vi "Main.vi"() -> ()   [LabVIEW 2013]
uses:
  Application Data.ctl
  State.ctl
panel:
  in  "Tahmin":i16
  in  "Tahmin Sayisi":u8=10 min=1
  in  "Tahmin Seç":bool
  out "Mesaj":string
  out "Bitti":bool
  out "Kalan":i16
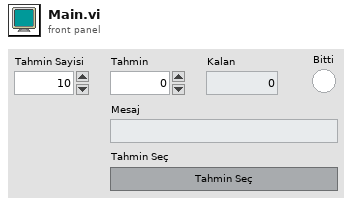
[diagram p1: front panel]
types:
  T1 = typedef "State.ctl" = enum16{"Initialise", "Make Guess", "Wait for event", "Sucess", "Fail", "End"}
  T2 = typedef "Application Data.ctl" = cluster{"Guesses Remaining":u8, "Guess":i16, "Message":string, "Correct":bool}
  T3 = enum8{"Enabled", "Disabled", "Disabled and Grayed Out"}
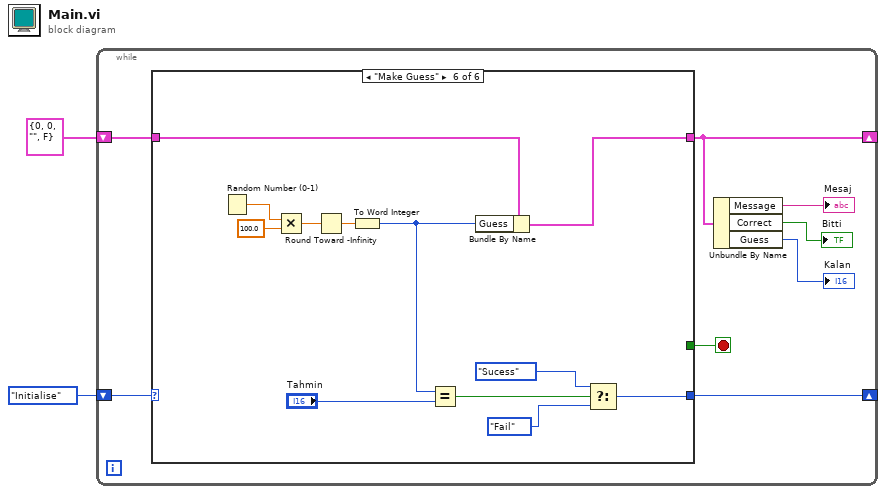
[diagram p0: block diagram]
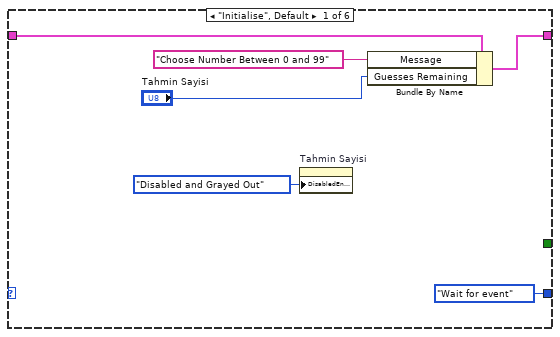
[diagram p2: hidden frame]
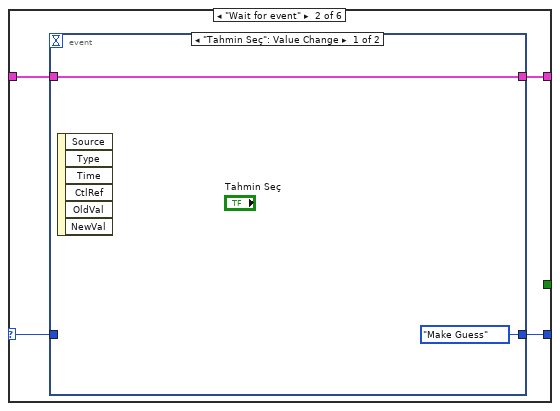
[diagram p3: hidden frame]
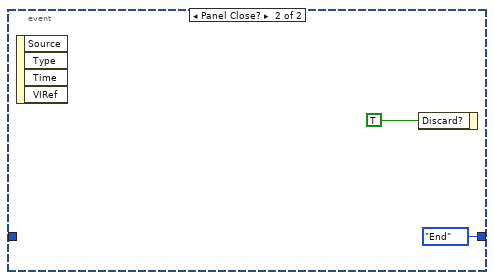
[diagram p4: hidden frame]
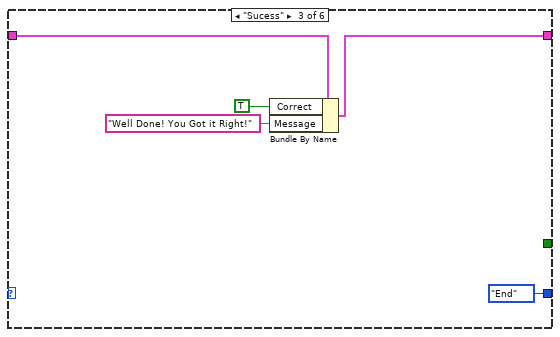
[diagram p5: hidden frame]
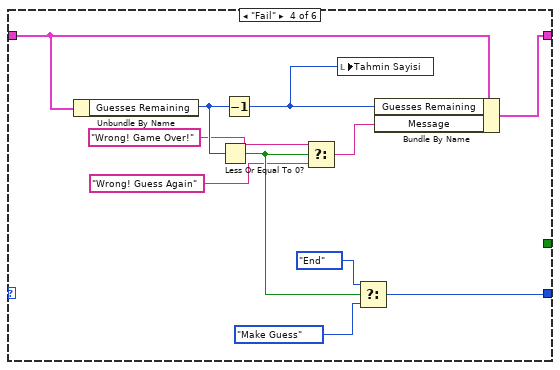
[diagram p6: hidden frame]
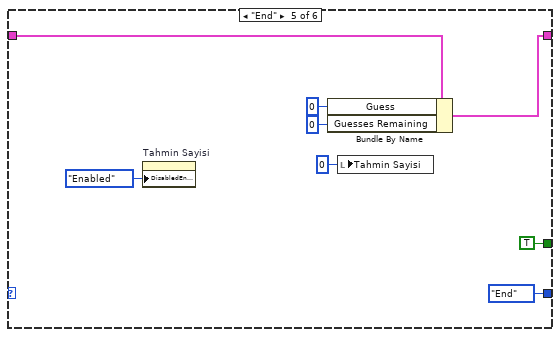
[diagram p7: hidden frame]
diagram:
  n1 = while {
    shift-right: [w9] -> _
    shift-left: T2 {"Guesses Remaining"=0, "Guess"=0, "Message"="", "Correct"=FALSE} ("Application Data") -> [w10]
    shift-right: [w7] -> _
    shift-left: State."Initialise" ("State") -> [w6]
    stop <- w5 stop-if-true
    n2 = case shown="\"Make Guess\"" w6 {
      selector: w6 -> [_ w17 _ _ _ _]
      tunnel: w10 -> [w16 w20 w29 w40 w45 w56]
      tunnel: [w15 w19 w28 w39 w44 w55] -> w9
      tunnel: [State."Wait for event" ("State") w18 State."End" ("State") w37 State."End" ("State") w49] -> w7
      tunnel: [_ _ _ _ TRUE _] -> w5
      frame "Initialise", Default {
        n3 = property on="Tahmin Sayisi" class="DigNum (strict)"("DisabledEnum"=T3."Disabled and Grayed Out" ("Disabled")) -> ()  [unwired: 2 in, 2 out]
        n4 = Bundle By Name(cluster=w16, "Message"="Choose Number Between 0 and 99", "Guesses Remaining"="Tahmin Sayisi") -> (w15:T2)
      }
      frame "Wait for event" {
        n5 = event shown="[0] \"Tahmin Seç\": Value Change" {
          selector: _ -> [_ _]
          dyn-events: _ -> [_ _]
          timeout: _ -> [_ _]
          tunnel: w20 -> [w22 _]
          tunnel: [w22 _] -> w19
          tunnel: [State."Make Guess" ("State") State."End" ("State")] -> w18
          tunnel: w17 -> [_ _]
          event "Tahmin Seç": Value Change {
            n6 = event-data() -> ()  [unwired: 1 in, 6 out]
          }
          event Panel Close? {
            n7 = event-data() -> ()  [unwired: 1 in, 4 out]
            n8 = event-data("Discard?"=TRUE) -> ()  [unwired: 1 in, 1 out]
          }
        }
      }
      frame "Sucess" {
        n9 = Bundle By Name(cluster=w29, "Correct"=TRUE, "Message"="Well Done! You Got it Right!") -> (w28:T2)
      }
      frame "Fail" {
        n10 = Unbundle By Name(w40) -> ("Guesses Remaining"=w38:u8)
        n11 = Less Or Equal To 0?(x=w38) -> (x <= 0?=w34:bool)
        n12 = Decrement(x=w38) -> (x-1=w30:u8)
        n13 = Select(t="Wrong! Game Over!", s=w34, f="Wrong! Guess Again") -> (s? t:f=w31:string)
        n14 = local write "Tahmin Sayisi"(w30) -> ()
        n15 = Select(t=State."End" ("State"), s=w34, f=State."Make Guess" ("State")) -> (s? t:f=w37:T1)
        n16 = Bundle By Name(cluster=w40, "Guesses Remaining"=w30, "Message"=w31) -> (w39:T2)
      }
      frame "End" {
        n17 = property on="Tahmin Sayisi" class="DigNum (strict)"("DisabledEnum"=T3."Enabled" ("Disabled")) -> ()  [unwired: 2 in, 2 out]
        n18 = Bundle By Name(cluster=w45, "Guess"=i16 0, "Guesses Remaining"=u8 0) -> (w44:T2)
        n19 = local write "Tahmin Sayisi"(u8 0 ("Tahmin Sayisi")) -> ()
      }
      frame "Make Guess" {
        n20 = Random Number (0-1)() -> (number: 0 to 1=w59:dbl)
        n21 = Multiply(x=w59, y=100.0) -> (x*y=w60:dbl)
        n22 = Round Toward -Infinity(1:w60) -> (0:w58:dbl)
        n23 = To Word Integer(number=w58) -> (16bit integer=w50:i16)
        n24 = Equal?(x=w50, y="Tahmin") -> (x = y?=w53:bool)
        n25 = Bundle By Name(cluster=w56, "Guess"=w50) -> (w55:T2)
        n26 = Select(t=State."Sucess" ("State"), s=w53, f=State."Fail" ("State")) -> (s? t:f=w49:T1)
      }
    }
    n27 = Unbundle By Name(w9) -> ("Message"=→"Mesaj":string, "Correct"=→"Bitti":bool, "Guess"=→"Kalan":i16)
  }
